vi "GT Set Laser Dis Table2D.vi"(0 "cardNum":i16, 1 "axisIndex":i16[](array[numeric])=[0, 0], 2 "count":i16[](array[numeric])=[0, 0], 3 "pRatio":dbl, 4 "pXPos":i32, 5 "pYPos":i32, 6 "minPower":dbl, 7 "error in (no error)":errorcluster caption="错误输入（无错误）", 8 "maxPower":dbl, 9 "pLimitPower":dbl, 10 "channel":i16) -> (19 "pLimitPower out":dbl, 20 "function return":i16, 21 "axisIndex out":i16[](array[numeric]), 22 "count out":i16[](array[numeric]), 23 "pRatio out":dbl, 24 "pXPos out":i32, 25 "pYPos out":i32, 27 "error out":errorcluster caption="错误输出")   [LabVIEW 2014, in "gts.lvlib"]
doc: "GT_API GT_SetLaserDisTable2D(short cardNum,short axisIndex[2],short count[2],double *pRatio,long *pXPos,long *pYPos, \n double minPower,double maxPower,double *pLimitPower,short channel=0);"
uses:
  gts.lvlib
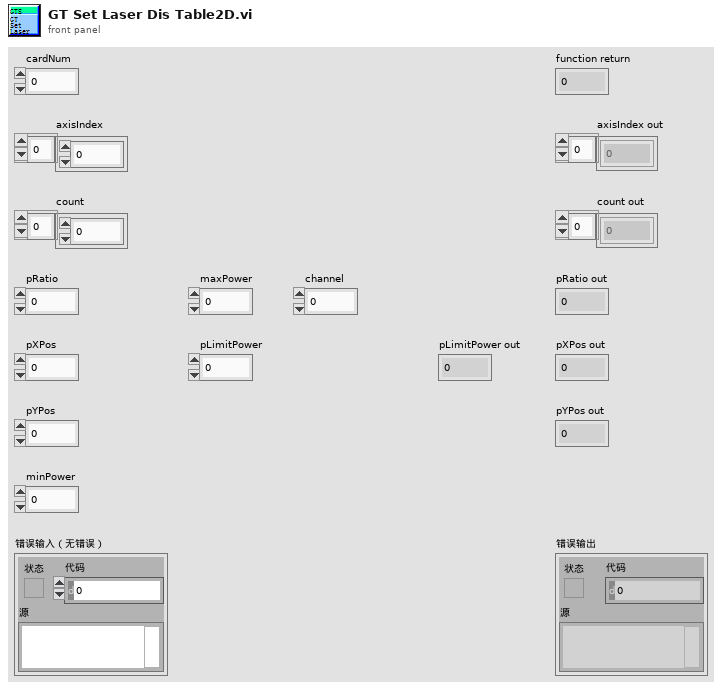
[diagram p1: front panel]
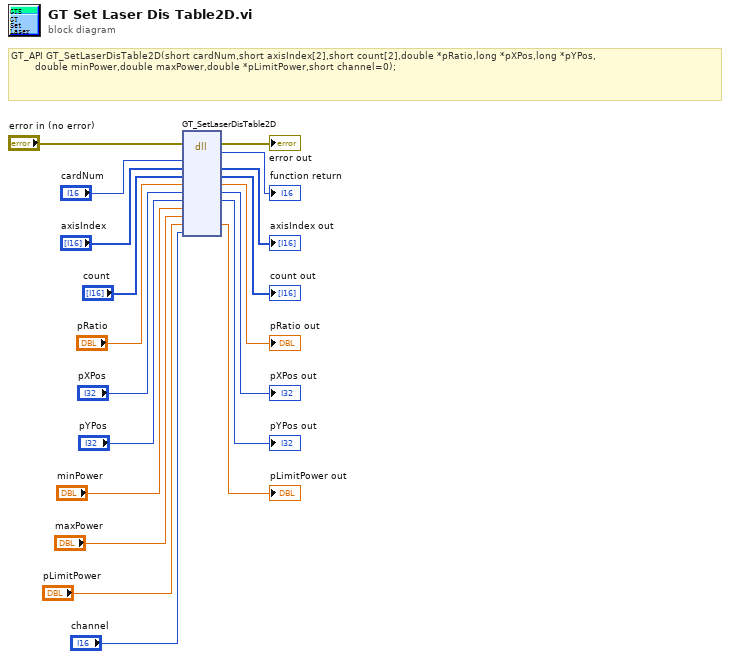
[diagram p0: block diagram]
diagram:
  # "GT_API GT_SetLaserDisTable2D(short cardNum,short axisIndex[2],short count[2],double *pRatio,long *pXPos,long *pYPos, \n\t\t\t\t\t\t\t double minPower,double maxPower,double *pLimitPower,short channel=0);"
  n1 = dll-call lib="PTH2habs D固高科技资料GTS控制卡GTS卡18年上半年资料dllVC32bit\nmulti_cardgts.*" fn="GT_SetLaserDisTable2D"(error in="error in (no error)", "cardNum"="cardNum", "axisIndex"="axisIndex", "count"="count", "pRatio"="pRatio", "pXPos"="pXPos", "pYPos"="pYPos", "minPower"="minPower", "maxPower"="maxPower", "pLimitPower"="pLimitPower", "channel"="channel") -> (error out=→"error out":errorcluster, →"function return":i16, "axisIndex"=→"axisIndex out":i16[], "count"=→"count out":i16[], "pRatio"=→"pRatio out":dbl, "pXPos"=→"pXPos out":i32, "pYPos"=→"pYPos out":i32, "pLimitPower"=→"pLimitPower out":dbl)  [unwired: 6 in, 1 out]
